vi "Read Message Length.vi"(8 "error in (no error)":errorcluster, 11 "TCP Listener in":refnum<class "TCP Listener.lvclass">) -> (0 "error out":errorcluster, 2 "Bytes to read":i32, 3 "TCP Listener out":refnum<class "TCP Listener.lvclass">)   [LabVIEW 2026, in "TALOS.lvlib" / "TCP Listener.lvlib" / "TCP Listener.lvclass"]
uses:
  TCP Listener.lvclass
  TCP Listener.lvclass/TCP Listener.ctl
  Support VIs/Global Constants.vi
  TALOS.lvlib
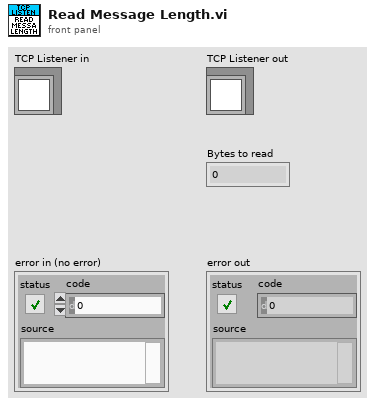
[diagram p1: front panel]
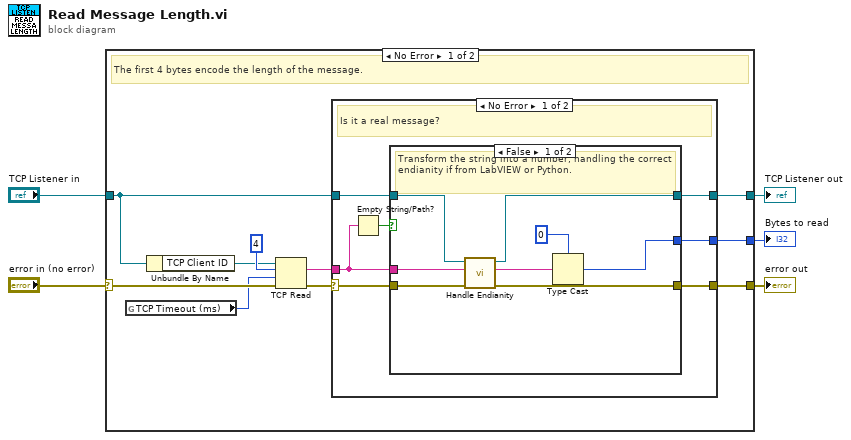
[diagram p0: block diagram]
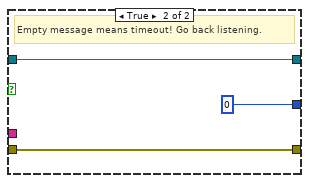
[diagram p2: hidden frame]
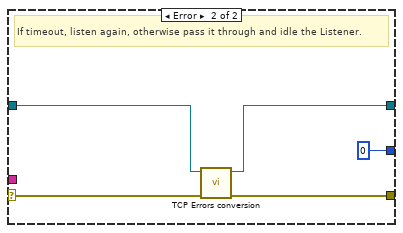
[diagram p3: hidden frame]
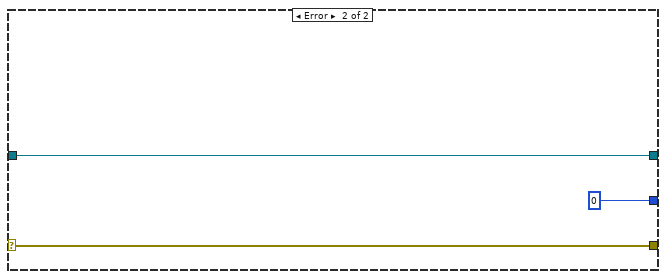
[diagram p4: hidden frame]
diagram:
  n1 = case shown="No Error" "error in (no error)" {
    selector: "error in (no error)" -> [w12 w40]
    tunnel: "TCP Listener in" -> [w8 w41]
    tunnel: [w15 w40] -> w4
    tunnel: [w10 w41] -> w2
    tunnel: [w9 0] -> w1
    frame No Error {
      # "The first 4 bytes encode the length of the message."
      n2 = global read "Global Constants.vi" "TCP Timeout (ms)"() -> (w6:i32)
      n3 = Unbundle By Name(w8) -> ("TCP Client ID"=w7:refnum<k5>)
      n4 = TCP Read(connection ID=w7, bytes to read=4, error in (no error)=w12, 9:w6) -> (data out=w14:string, error out=w13:errorcluster)  [unwired: 1 in, 1 out]
      n5 = case shown="No Error" w13 {
        selector: w13 -> [w21 w38]
        tunnel: w14 -> [w16 _]
        tunnel: [w17 w36] -> w15
        tunnel: w8 -> [w20 w37]
        tunnel: [w19 w35] -> w10
        tunnel: [w18 0] -> w9
        frame No Error {
          # "Is it a real message?"
          n6 = Empty String/Path?(string/path=w16) -> (empty?=w22:bool)
          n7 = case shown="False" w22 {
            tunnel: w21 -> [w28 w32]
            tunnel: w20 -> [w30 w33]
            tunnel: [w25 w33] -> w19
            tunnel: [w24 0] -> w18
            tunnel: [w27 w32] -> w17
            tunnel: w16 -> [w29 _]
            frame False {
              # "Transform the string into a number, handling the correct endianity if from LabVIEW or Python."
              n8 = call-dynamic "Handle Endianity.vi"("error in (no error)"=w28, "Byte to read in"=w29, "TCP Listener in"=w30) -> ("error out"=w27:errorcluster, "Bytes to read out"=w26:string, "TCP Listener out"=w25:refnum<class "TCP Listener.lvclass">)  [unwired: 6 in]
              n9 = Type Cast(type=0, x=w26) -> (*(type *) &x=w24:i32)
            }
            frame True {
              # "Empty message means timeout! Go back listening."
            }
          }
        }
        frame Error {
          # "If timeout, listen again, otherwise pass it through and idle the Listener."
          n10 = call-dynamic "TCP Errors conversion.vi"("error in (no error)"=w38, "TCP Listener in"=w37) -> ("error out"=w36:errorcluster, "TCP Listener out"=w35:refnum<class "TCP Listener.lvclass">)  [unwired: 8 in]
        }
      }
    }
    frame Error {
    }
  }
  "error out" <- w4
  "TCP Listener out" <- w2
  "Bytes to read" <- w1
